vi "Is Actor Stop Error.vi"(1 "error in":errorcluster) -> (0 "Stop Error":bool)   [LabVIEW 2016, in "_Parent Actor Template.lvlib" / "_Parent Actor Template.lvclass"]
uses:
  _Parent Actor Template.lvclass
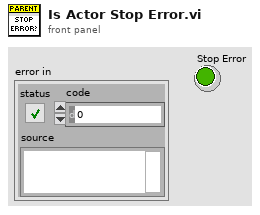
[diagram p1: front panel]
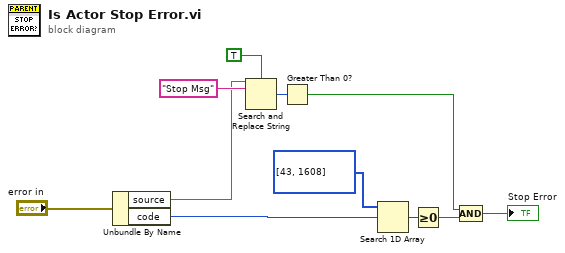
[diagram p0: block diagram]
diagram:
  n1 = Unbundle By Name("error in") -> ("source"=w5:string, "code"=w9:i32)
  n2 = Search and Replace String(case sensitive?=TRUE ("ignore case? (F)"), input string=w5, search string="Stop Msg") -> (number of replacements=w8:i32)  [unwired: 5 in, 3 out]
  n3 = Greater Than 0?(x=w8) -> (x > 0?=w2:bool)
  n4 = Search 1D Array(1D array=i32[] [43, 1608], element=w9) -> (index of element=w11:i32)  [unwired: 1 in]
  n5 = Greater Or Equal To 0?(x=w11) -> (x >= 0?=w3:bool)
  n6 = Compound Arithmetic op=AND(w2, w3) -> (→"Stop Error":bool)
